vi "YAML Get Field Value Bool.vi"(10 "field name":string, 11 "array of strings":string[][](array[string])) -> (2 "Boolean":bool)   [LabVIEW 2011]
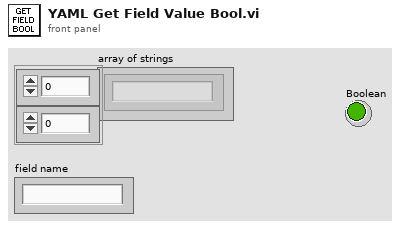
[diagram p1: front panel]
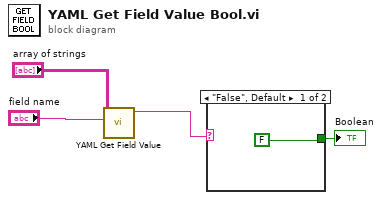
[diagram p0: block diagram]
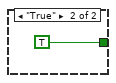
[diagram p2: hidden frame]
diagram:
  n1 = call "YAML Get Field Value.vi"("field name"="field name", "array of strings"="array of strings") -> ("field value"=w2:string)  [unwired: 9 in]
  n2 = case shown="\"False\", Default" w2 {
    tunnel: [FALSE TRUE] -> w1
    frame "False", Default {
    }
    frame "True" {
    }
  }
  "Boolean" <- w1
